vi "Parse Response and Report Error.vi"(8 "error in (no error)":errorcluster, 10 "Parameter":string, 11 "Response string":string) -> (0 "error out":errorcluster, 3 "Value Out":dbl format="%.4g")   [LabVIEW 2020, in "PS Driver.lvlib" / "PS Driver AMI4xx.lvclass"]
uses:
  PS Driver AMI4xx.lvclass
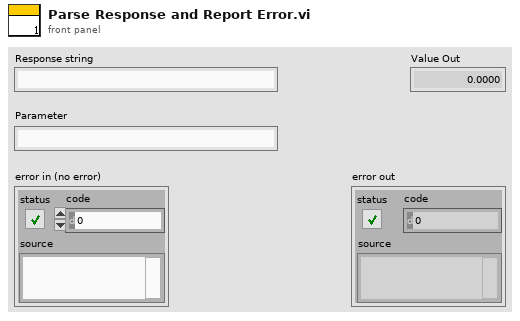
[diagram p1: front panel]
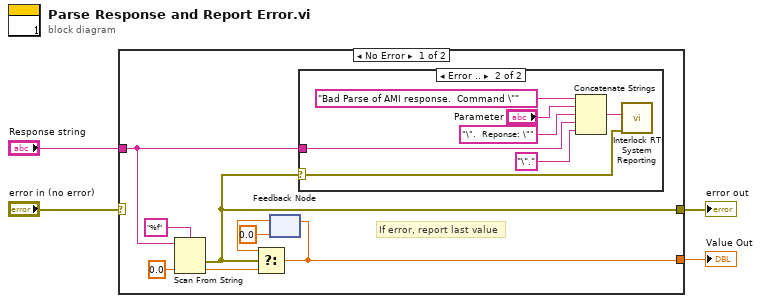
[diagram p0: block diagram]
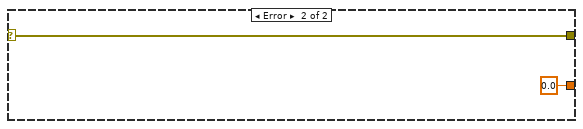
[diagram p3: hidden frame]
diagram:
  n1 = case shown="No Error" "error in (no error)" {
    selector: "error in (no error)" -> [_ w21]
    tunnel: "Response string" -> [w10 _]
    tunnel: [w7 0.0 ("default value 1")] -> w3
    tunnel: [w5 w21] -> w2
    frame No Error {
      # "If error, report last value"
      n2 = Scan From String(format string="%f", input string=w10, default 1=0.0 ("default value 1")) -> (error out=w5:errorcluster, output 1=w9:dbl)  [unwired: 2 in, 2 out]
      n3 = feedback #1(0.0) -> (w8:dbl)
      n4 = Select(t=w8, s=w5, f=w9) -> (s? t:f=w7:dbl)
      n5 = feedback-in #1(w7) -> ()
      n6 = case shown="Error .." w5 {
        selector: w5 -> [_ w13]
        tunnel: w10 -> [_ w15]
        frame No Error {
        }
        frame Error {
          n7 = Concatenate Strings("Bad Parse of AMI response.  Command \"" ("format string"), "Parameter", "\".  Reponse: \"" ("format string"), w15, "\"." ("format string")) -> (w14:string)
          n8 = call "Interlock RT System Reporting.vi"("Error In"=w13, "String"=w14) -> ()  [unwired: 8 in, 2 out]
        }
      }
    }
    frame Error {
    }
  }
  "Value Out" <- w3
  "error out" <- w2
